vi "Write Multiple Coils.vi"(8 "error in (no error)":errorcluster, 9 "values":bool[](array[boolean]), 10 "address":u16, 11 "MODBUS in":refnum<class "Modbus.lvclass">) -> (0 "error out":errorcluster, 3 "MODBUS Out":refnum<class "Modbus.lvclass">)   [LabVIEW 2020, in "Library Instrument & Equipement.lvlib" / "Library Relay_Board.lvlib" / "Modbus.lvclass"]
doc: "Writes multiple coil <B>values</B> starting at specified <B>address</B> (Modbus function code: <B>15</B>)."
uses:
  Modbus.lvclass
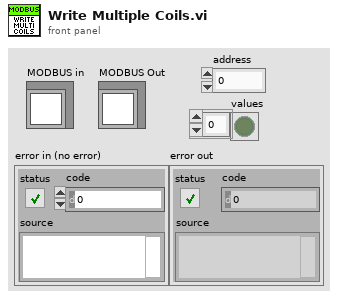
[diagram p1: front panel]
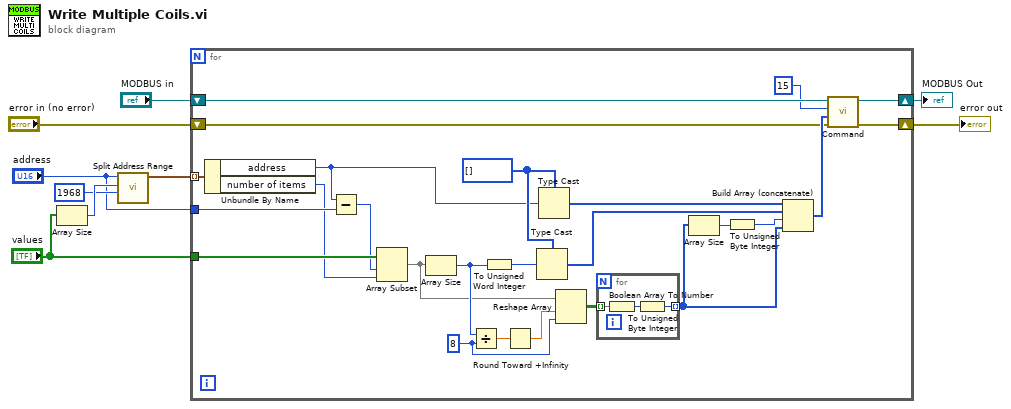
[diagram p0: block diagram]
diagram:
  n1 = Array Size(array="values") -> (size(s)=w6:i32)
  n2 = call "Split Address Range.vi"("max number of items"=u16 1968, "number of items"=w6, "address"="address") -> ("addresses and numbers of items"=w4:cluster{"address":u16, "number of items":u16}[])  [unwired: 8 in]
  n3 = for {
    tunnel: "values" -> [w13]
    shift-right: [w28] -> w8
    shift-left: "MODBUS in" -> [w34]
    shift-right: [w26] -> w1
    shift-left: "error in (no error)" -> [w27]
    tunnel: w4 -> [w16] mode=indexing
    tunnel: "address" -> [w14]
    w22 = 8 ("y")
    w33 = u8[] []
    n4 = Unbundle By Name(w16) -> ("address"=w15:u16, "number of items"=w10:u16)
    n5 = Subtract(x=w15, y=w14) -> (x-y=w11:u16)
    n6 = Array Subset(array=w13, index=w11, length=w10) -> (w12:bool[])
    n7 = Array Size(array=w12) -> (size(s)=w20:i32)
    n8 = Divide(x=w20, y=w22) -> (x/y=w24:dbl)
    n9 = To Unsigned Word Integer(number=w20) -> (unsigned 16bit integer=w25:u16)
    n10 = Round Toward +Infinity(x=w24) -> (ceil(x): smallest int >= x=w23:dbl)
    n11 = Type Cast(type=w33, x=w25) -> (*(type *) &x=w31:u8[])
    n12 = Type Cast(type=w33, x=w15) -> (*(type *) &x=w32:u8[])
    n13 = Reshape Array(w12, w23, w22) -> (w21:bool[][])
    n14 = for {
      tunnel: w21 -> [w37] mode=indexing
      tunnel: [w35] -> w18 mode=indexing
      n15 = Boolean Array To Number(Boolean array=w37) -> (number=w36:u32)
      n16 = To Unsigned Byte Integer(number=w36) -> (unsigned 8bit integer=w35:u8)
    }
    n17 = Array Size(array=w18) -> (size(s)=w19:i32)
    n18 = To Unsigned Byte Integer(number=w19) -> (unsigned 8bit integer=w17:u8)
    n19 = Build Array (concatenate)(w32, w31, w17, w18) -> (w30:u8[])
    n20 = call-dynamic "Command.vi"("error in (no error)"=w27, "data in"=w30, "function code"=u8 15 ("function"), "MODBUS in"=w34) -> ("error out"=w26:errorcluster, "MODBUS Out"=w28:refnum<class "Modbus.lvclass">)  [unwired: 5 in, 1 out]
  }
  "MODBUS Out" <- w8
  "error out" <- w1
